vi "Viewer.vi"(4 "Col Array Refnum":refnum<vi>, 5 "RepoPath Refnum":refnum<vi>, 6 "SetList Layout Ref":refnum<vi>, 7 "GitCmd Refnum":refnum<vi>, 8 "SetList Dev queue":refnum<queue>, 9 "SetList VariableManager ref":refnum<vi>, 10 "SetList Clipboard ref":refnum<vi>) -> ()   [LabVIEW 2013]
doc: "View read-only procedure (table, variables, functions, device setup). Copy values from viewer into SetList via input references."
uses:
  DeviceVIs/Device/Device.lvclass
  ColumnVIs/Column/Column.lvclass
  VariableManagerCodes/VariableManager/VariableManager.lvclass
  <vilib>/Utility/miscctls.llb/LVRowAndColumnTypeDef.ctl
  VariableManagerCodes/API/VariableManagerAPI.lvlib
panel:
  in  "LoadFromRepo":bool
  out "SetList Procedure Description":string
  out "SetList Hash":string
  out "Invalid ref Warning":string="LOST LINK TO SetList:\nPlease close this window and relaunch from SetList."
  out "SetList Procedure Name":string
  out "SetList Version":string
  in  "Tab Control":T1(tab)
  in  "Layouts2SetList Button":bool
  in  "FitCol2Text Button":bool
  in  "View Devices Button":bool
  in  "Select Layout":i32(ring)=-1 items=["(On-the-fly)"=-2, "All"=-1]
  in  "Viewer Table":string[][](table)=[["", "", "Ramp", "1", "0.1", "0", "0", "0", "0", "0", "0", "0", "0", "0", "0", "0", "0", "0", "0", "0", "0", "0", "0", "0", "0", "0", "0", "0", "0", "0"]]
  out "Useful Functions":string="-- not functionality for strings (always treated as double)\nfunction bnot(a)\n   -- this \"(bool exp.) and b or c\" is equivalent to \"(bool exp.) ? b : c\" syntax.\n   -- caution: undefined variables evaluate to \"false\" so will NOT throw an error as argument\n   return a==0 and 1 or 0\nend"
  out "Viewer: User Functions":string
  out "RepoPath?":bool
  out "GitCmd?":bool
  out "SetList Col Array?":bool
  out "SetList Layout Ring?":bool
  out "SetList Dev queue?":bool
  out "SetList Variables?\n(on startup only)":bool
  out "SetList Clipboard?":bool
  in  "Viewer VariableManager.lvclass":refnum<class "VariableManager.lvclass">
  out "View Dev queue":refnum<queue>
  out "View Col array":refnum<class "Column.lvclass">[](array[class])
  in  "Devices":refnum<class "Device.lvclass">[](array[class])
  out "Mouse Down on header":bool
  # "SetList Viewer (Read-only)"
  # "In the context of ramps several variables are passed or specified that may be used here:\n\n   - f the fractional position of a point in a ramp\n   - t the current time in a ramp\n   - dt the current timestep size.\n   - tMax the total duration of the ramp"
  # "Invalid reference?"
  # "SetList references"
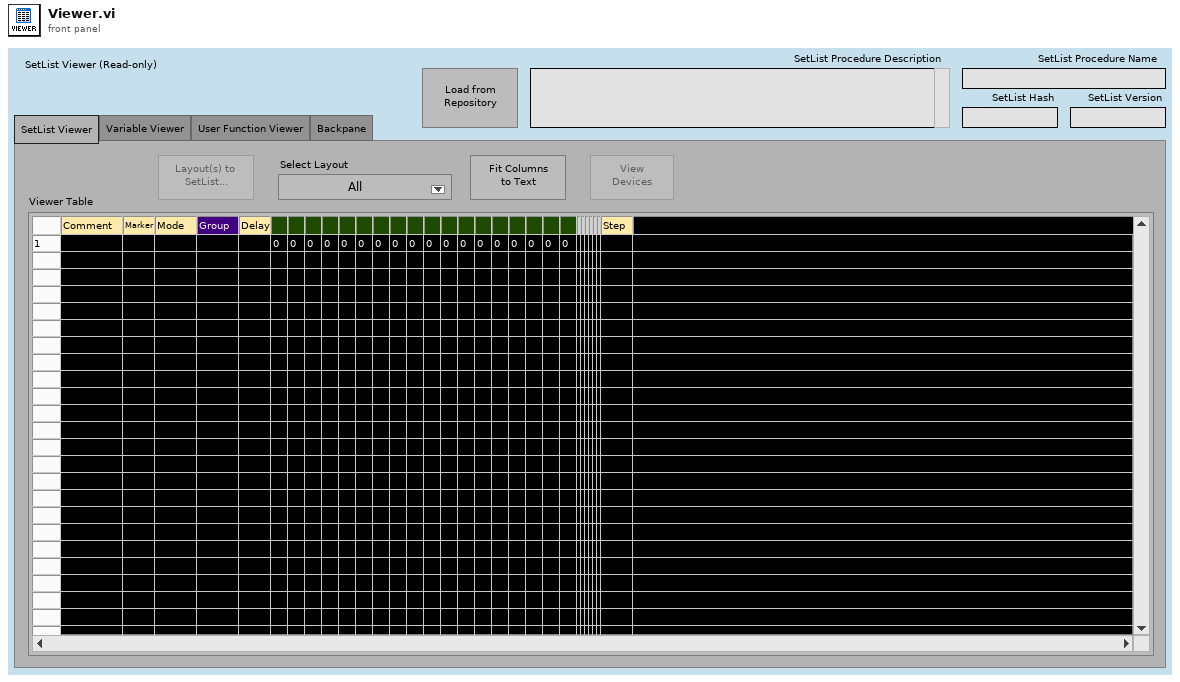
[diagram p1: front panel]
types:
  T1 = enum32{"SetList Viewer", "Variable Viewer", "User Function Viewer", "Backpane"}
  T2 = typedef "LVRowAndColumnTypeDef.ctl" = cluster{"Row":i32, "Column":i32}
  T3 = enum8{"Enabled", "Disabled", "Disabled and Grayed Out"}
  T4 = typedef "SaveCluster.ctl" = cluster{"Version":string, "Devices":refnum<class "Device.lvclass">[], "Select Layout":i32, "Layout:Strings And Values []":T5, "User defined functions":string, "VariableManager":refnum<class "VariableManager.lvclass">}
  T5 = typedef "LVStringsAndValuesArrayTypeDef_I32.ctl" = cluster{"String":string, "Value":i32}[]
  T6 = typedef "CommitCluster.ctl" = cluster{"Hash":string, "Date":string, "Name":string}
  T7 = typedef "LVPoint32TypeDef.ctl" = cluster{"Horizontal":i32, "Vertical":i32}
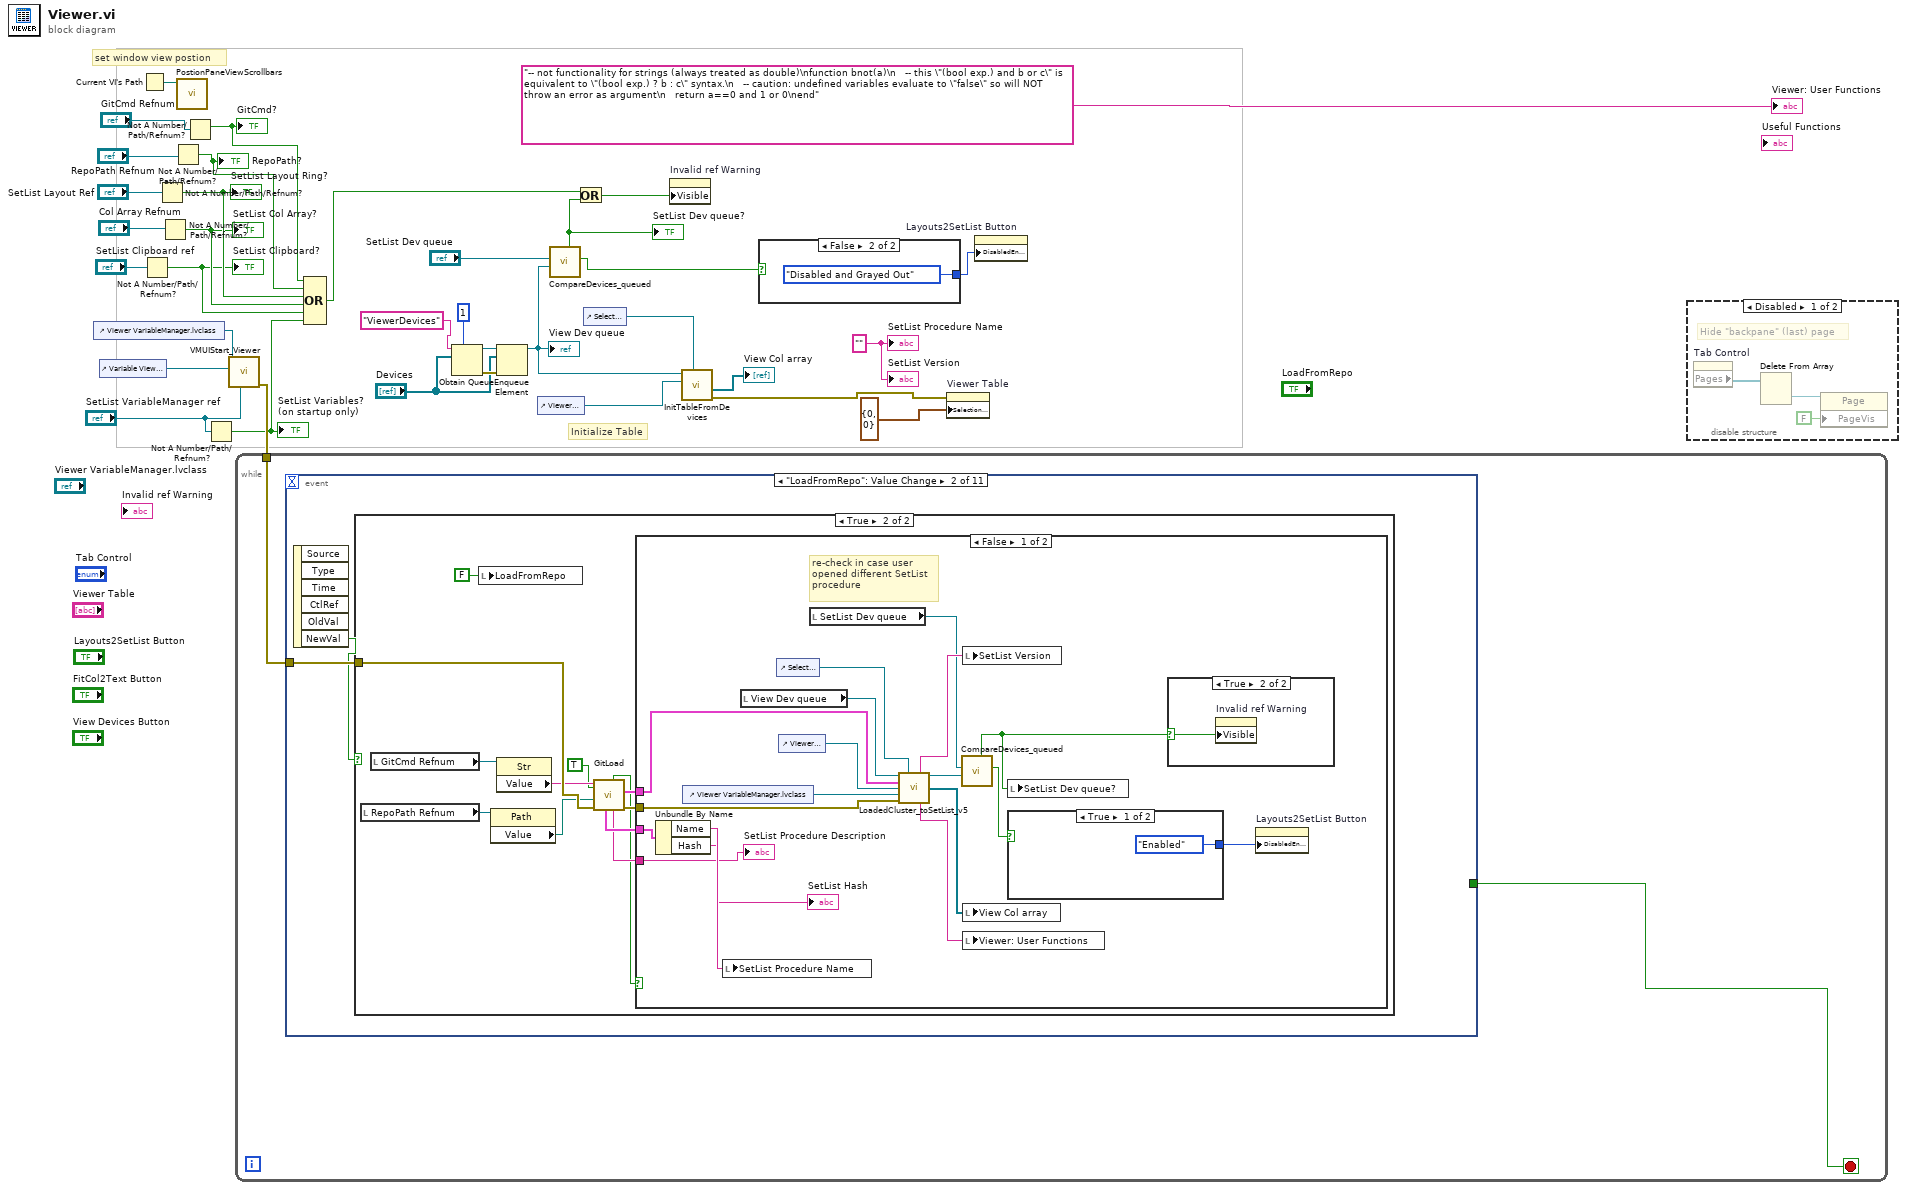
[diagram p0: block diagram]
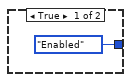
[diagram p2: hidden frame]
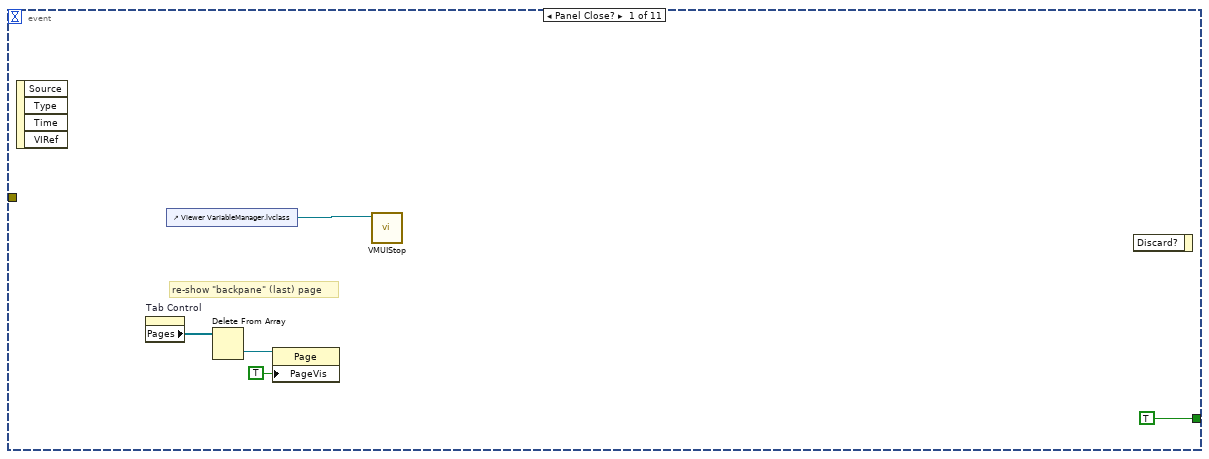
[diagram p4: hidden frame]
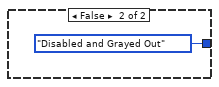
[diagram p7: hidden frame]
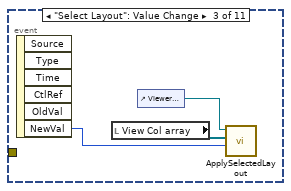
[diagram p9: hidden frame]
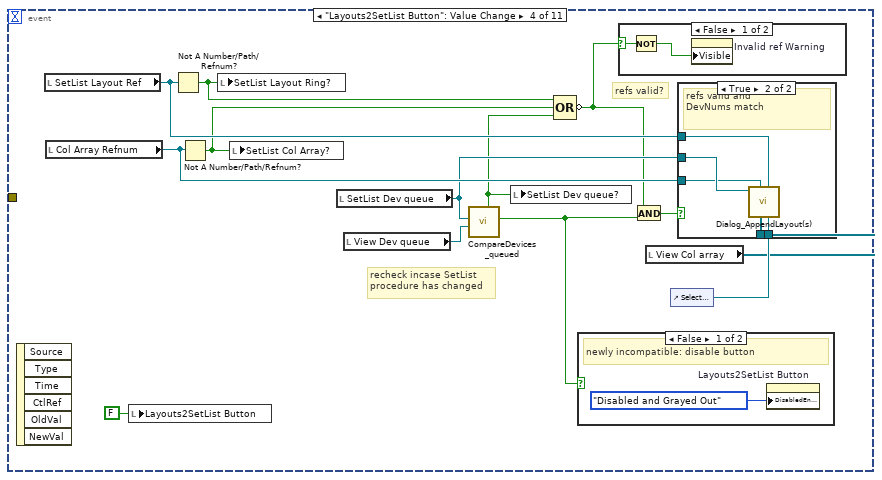
[diagram p10: hidden frame]
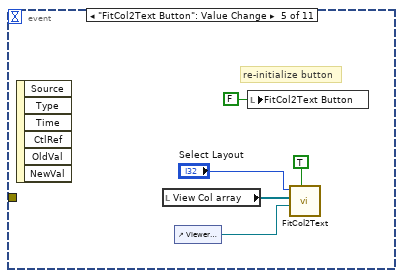
[diagram p14: hidden frame]
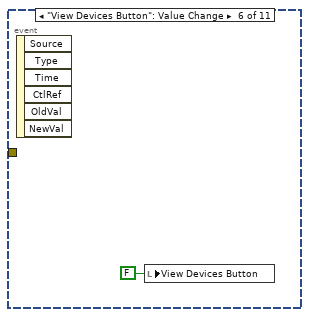
[diagram p15: hidden frame]
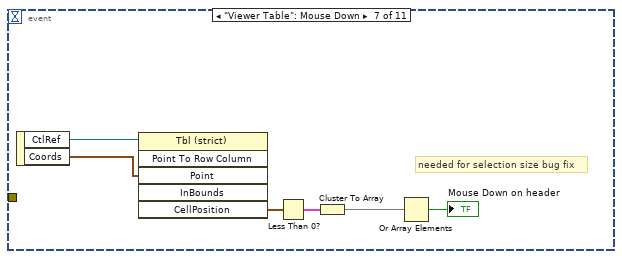
[diagram p16: hidden frame]
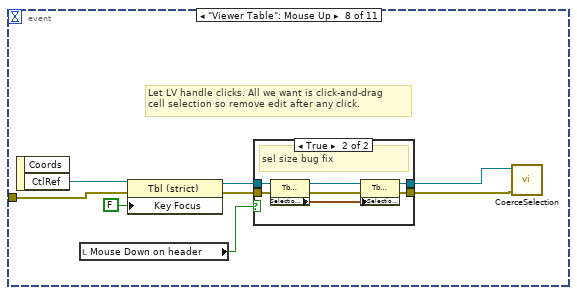
[diagram p17: hidden frame]
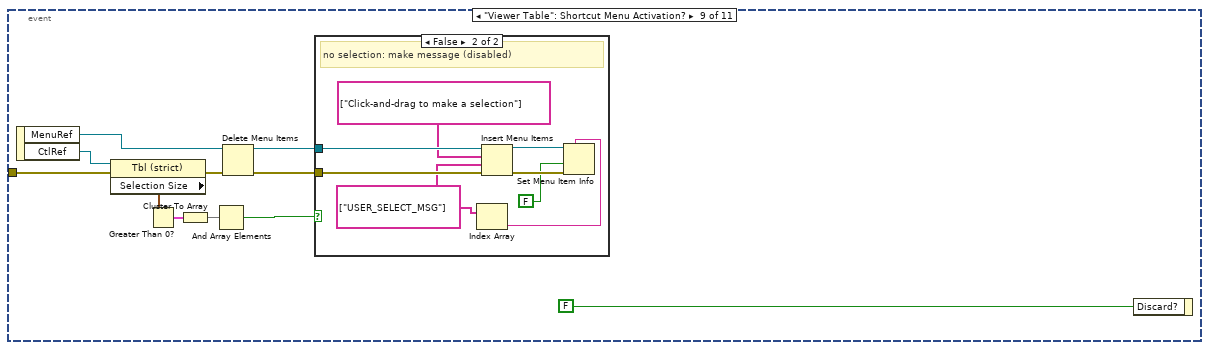
[diagram p19: hidden frame]
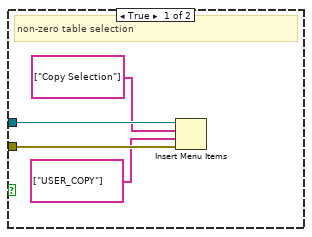
[diagram p20: hidden frame]
diagram:
  w27 = "" ("SetList Procedure Name")
  # "set window view postion"
  # "Initialize Table"
  n1 = control-ref of="Viewer VariableManager.lvclass"() -> (w24:refnum<vi>)
  n2 = control-ref of="Variable View Pane"() -> (w25:refnum<vi>)
  n3 = Current VI's Path() -> (path=w18:path)
  n4 = Not A Number/Path/Refnum?(number/path/refnum="SetList Clipboard ref") -> (NaN/Path/Refnum?=w13:bool)
  "SetList Clipboard?" <- w13
  n5 = Not A Number/Path/Refnum?(number/path/refnum="SetList Layout Ref") -> (NaN/Path/Refnum?=w15:bool)
  "SetList Layout Ring?" <- w15
  n6 = Not A Number/Path/Refnum?(number/path/refnum="Col Array Refnum") -> (NaN/Path/Refnum?=w14:bool)
  "SetList Col Array?" <- w14
  n7 = Not A Number/Path/Refnum?(number/path/refnum="RepoPath Refnum") -> (NaN/Path/Refnum?=w1:bool)
  "RepoPath?" <- w1
  n8 = call "PostionPaneViewScrollbars.vi"("vi path"=w18) -> ()  [unwired: 10 in, 1 out]
  n9 = Not A Number/Path/Refnum?(number/path/refnum="GitCmd Refnum") -> (NaN/Path/Refnum?=w2:bool)
  "GitCmd?" <- w2
  n10 = Not A Number/Path/Refnum?(number/path/refnum="SetList VariableManager ref") -> (NaN/Path/Refnum?=w12:bool)
  "SetList Variables?\n(on startup only)" <- w12
  n11 = call "VMUIStart_Viewer.vi"("SetList VariableManager Ref in"="SetList VariableManager ref", "SubPanelRef"=w25, "Viewer VariableManager Ref in"=w24) -> ("error out"=w23:errorcluster)  [unwired: 7 in, 1 out]
  n12 = while {
    tunnel: w23 -> [w36]
    stop <- w37 stop-if-true
    n13 = event shown="[1] \"LoadFromRepo\": Value Change" {
      selector: _ -> [_ _ _ _ _ _ _ _ _ _ _]
      dyn-events: _ -> [_ _ _ _ _ _ _ _ _ _ _]
      timeout: _ -> [_ _ _ _ _ _ _ _ _ _ _]
      tunnel: [TRUE ("true") _ _ _ _ _ _ _ _ _ _] -> w37
      tunnel: w36 -> [_ w44 _ _ _ _ _ w120 w141 w155 _]
      event Panel Close? {
        # "re-show \"backpane\" (last) page"
        n14 = event-data() -> ()  [unwired: 1 in, 4 out]
        n15 = property on="Tab Control" class="TabCtl (strict)"() -> ("Pages"=w40:refnum<vi>[])  [unwired: 2 in, 2 out]
        n16 = control-ref of="Viewer VariableManager.lvclass"() -> (w41:refnum<vi>)
        n17 = Delete From Array(array=w40) -> (deleted portion=w39:refnum<vi>)  [unwired: 2 in, 1 out]
        n18 = property class="Page"(reference=w39, "PageVis"=TRUE ("Page Visible")) -> ()  [unwired: 1 in, 2 out]
        n19 = call "VMUIStop.vi"("VariableManagerRef in"=w41) -> ()  [unwired: 9 in, 2 out]
        n20 = event-data() -> ()  [unwired: 2 in, 1 out]
      }
      event "LoadFromRepo": Value Change {
        n21 = event-data() -> ("NewVal"=w43:bool)  [unwired: 1 in, 5 out]
        n22 = case shown="True" w43 {
          tunnel: w44 -> [_ w54]
          frame False {
          }
          frame True {
            n23 = local read "RepoPath Refnum"() -> (w50:refnum<vi>)
            n24 = local read "GitCmd Refnum"() -> (w52:refnum<vi>)
            n25 = local write "LoadFromRepo"(FALSE ("LoadFromRepo")) -> ()
            n26 = property class="Path"(reference=w50) -> ("Value"=w49:path)  [unwired: 1 in, 2 out]
            n27 = property class="Str"(reference=w52) -> ("Value"=w51:string)  [unwired: 1 in, 2 out]
            n28 = call "GitLoad.vi"("Viewer?"=TRUE, "error in (no error)"=w54, "Directory"=w49, "Git exec"=w51) -> ("error out"=w55:errorcluster, "Save Cluster"=w56:T4, "Loaded Description"=w47:string, "User Cancelled"=w45:bool, "Loaded Commit Info"=w53:T6)  [unwired: 1 in, 2 out]
            n29 = case shown="False" w45 {
              tunnel: w56 -> [w62 _]
              tunnel: w55 -> [w61 _]
              tunnel: w53 -> [w60 _]
              tunnel: w47 -> [w58 _]
              frame False {
                # "re-check in case user\nopened different SetList\nprocedure"
                n30 = Unbundle By Name(w60) -> ("Name"=w59:string, "Hash"=→"SetList Hash":string)
                n31 = control-ref of="Viewer VariableManager.lvclass"() -> (w69:refnum<vi>)
                n32 = local write "SetList Procedure Name"(w59) -> ()
                n33 = local read "View Dev queue"() -> (w65:refnum<queue>)
                n34 = control-ref of="Select Layout"() -> (w74:refnum<vi>)
                n35 = control-ref of="Viewer Table"() -> (w73:refnum<vi>)
                n36 = local read "SetList Dev queue"() -> (w67:refnum<queue>)
                n37 = call "LoadedCluster_toSetList_v5.vi"("Devices queue"=w65, "Layout Ref"=w74, "Save Cluster"=w62, "Table Ref in"=w73, "VariableManagerRef"=w69, "error in (no error)"=w61) -> ("Loaded Version"=w72:string, "Devices queue out"=w63:refnum<queue>, "Col array"=w71:refnum<class "Column.lvclass">[], "User defined functions"=w70:string)  [unwired: 4 in, 2 out]
                n38 = call "CompareDevices_queued.vi"("New Dev queue"=w63, "Old Dev queue"=w67) -> ("compatible?"=w66:bool, "Old Dev queue invalid?"=w64:bool)  [unwired: 7 in, 1 out]
                n39 = local write "SetList Version"(w72) -> ()
                n40 = local write "View Col array"(w71) -> ()
                n41 = local write "Viewer: User Functions"(w70) -> ()
                n42 = local write "SetList Dev queue?"(w64) -> ()
                n43 = case shown="True" w66 {
                  tunnel: [T3."Enabled" ("Disabled") T3."Disabled and Grayed Out" ("Disabled")] -> w68
                  frame True {
                  }
                  frame False {
                  }
                }
                n44 = case shown="True" w64 {
                  selector: w64 -> [_ w75]
                  frame False {
                  }
                  frame True {
                    n45 = property on="Invalid ref Warning" class="Str"("Visible"=w75) -> ()  [unwired: 2 in, 2 out]
                  }
                }
                n46 = property on="Layouts2SetList Button" class="Bool (strict)"("DisabledEnum"=w68) -> ()  [unwired: 2 in, 2 out]
                "SetList Procedure Description" <- w58
              }
              frame True {
              }
            }
          }
        }
      }
      event "Select Layout": Value Change {
        n47 = event-data() -> ("NewVal"=w80:i32)  [unwired: 1 in, 5 out]
        n48 = local read "View Col array"() -> (w79:refnum<class "Column.lvclass">[])
        n49 = control-ref of="Viewer Table"() -> (w78:refnum<vi>)
        n50 = call "ApplySelectedLayout.vi"("Layout index"=w80, "Col array"=w79, "Tbl Refnum"=w78) -> ()  [unwired: 8 in, 1 out]
      }
      event "Layouts2SetList Button": Value Change {
        # "recheck incase SetList\nprocedure has changed"
        # "refs valid?"
        n51 = event-data() -> ()  [unwired: 1 in, 6 out]
        n52 = local read "SetList Layout Ref"() -> (w91:refnum<vi>)
        n53 = local read "Col Array Refnum"() -> (w86:refnum<vi>)
        n54 = local write "Layouts2SetList Button"(FALSE ("Layouts2SetList Button")) -> ()
        n55 = Not A Number/Path/Refnum?(number/path/refnum=w91) -> (NaN/Path/Refnum?=w90:bool)
        n56 = Not A Number/Path/Refnum?(number/path/refnum=w86) -> (NaN/Path/Refnum?=w87:bool)
        n57 = local write "SetList Layout Ring?"(w90) -> ()
        n58 = local write "SetList Col Array?"(w87) -> ()
        n59 = local read "SetList Dev queue"() -> (w84:refnum<queue>)
        n60 = local read "View Dev queue"() -> (w85:refnum<queue>)
        n61 = call "CompareDevices_queued.vi"("New Dev queue"=w85, "Old Dev queue"=w84) -> ("compatible?"=w82:bool, "Old Dev queue invalid?"=w83:bool)  [unwired: 7 in, 1 out]
        n62 = local write "SetList Dev queue?"(w83) -> ()
        n63 = Compound Arithmetic op=OR(w90, w87, w83) -> (invert w81:bool)
        n64 = case shown="False" w82 {
          frame False {
            # "newly incompatible: disable button"
            n65 = property on="Layouts2SetList Button" class="Bool (strict)"("DisabledEnum"=T3."Disabled and Grayed Out" ("Disabled")) -> ()  [unwired: 2 in, 2 out]
          }
          frame True {
          }
        }
        n66 = case shown="False" w81 {
          selector: w81 -> [w95 _]
          frame False {
            n67 = Not(x=w95) -> (.not. x?=w94:bool)
            n68 = property on="Invalid ref Warning" class="Str"("Visible"=w94) -> ()  [unwired: 2 in, 2 out]
          }
          frame True {
          }
        }
        n69 = And(x=w81, y=w82) -> (x .and. y?=w92:bool)
        n70 = local read "View Col array"() -> (w88:refnum<class "Column.lvclass">[])
        n71 = control-ref of="Select Layout"() -> (w89:refnum<vi>)
        n72 = case shown="True" w92 {
          tunnel: w91 -> [_ w101]
          tunnel: w84 -> [_ w98]
          tunnel: w89 -> [_ w100]
          tunnel: w88 -> [_ w99]
          tunnel: w86 -> [_ w97]
          frame False {
            # "refs inalid or\nDevNum mis-match"
          }
          frame True {
            # "refs valid and \nDevNums match"
            n73 = call "Dialog_AppendLayout(s).vi"("Viewer Layout Ref"=w100, "SetList Layout Ref"=w101, "View Col array"=w99, "Col Array Refnum"=w97, "SetList Dev queue"=w98) -> ()  [unwired: 7 in]
          }
        }
      }
      event "FitCol2Text Button": Value Change {
        # "re-initialize button"
        n74 = event-data() -> ()  [unwired: 1 in, 6 out]
        n75 = local read "View Col array"() -> (w106:refnum<class "Column.lvclass">[])
        n76 = control-ref of="Viewer Table"() -> (w103:refnum<vi>)
        n77 = local write "FitCol2Text Button"(FALSE ("FitCol2Text Button")) -> ()
        n78 = call "FitCol2Text.vi"("Defer Updates?"=TRUE, "SetList Table ref"=w103, "Col array"=w106, "Select Layout"="Select Layout") -> ()  [unwired: 7 in, 1 out]
      }
      event "View Devices Button": Value Change {
        n79 = event-data() -> ()  [unwired: 1 in, 6 out]
        n80 = local write "View Devices Button"(FALSE ("View Devices Button")) -> ()
      }
      event "Viewer Table": Mouse Down {
        # "needed for selection size bug fix"
        n81 = event-data() -> ("CtlRef"=w113:refnum<vi>, "Coords"=w112:T7)  [unwired: 1 in]
        n82 = invoke on="Invoke Node" class="Tbl (strict)" method="Point To Row Column"(reference=w113, "Point"=w112) -> ("CellPosition"=w111:T2)  [unwired: 4 in, 5 out]
        n83 = Less Than 0?(x=w111) -> (x < 0?=w110:cluster{"Row":bool, "Column":bool})
        n84 = Cluster To Array(cluster=w110) -> (array=w109:bool[])
        n85 = Or Array Elements(Boolean array=w109) -> (logical OR=→"Mouse Down on header":bool)
      }
      event "Viewer Table": Mouse Up {
        # "Let LV handle clicks. All we want is click-and-drag\ncell selection so remove edit after any click."
        n86 = event-data() -> ("CtlRef"=w121:refnum<vi>)  [unwired: 1 in, 1 out]
        n87 = local read "Mouse Down on header"() -> (w114:bool)
        n88 = property class="Tbl (strict)"(reference=w121, error in=w120, "Key Focus"=FALSE) -> (reference out=w118:refnum<vi>, error out=w116:errorcluster)
        n89 = case shown="True" w114 {
          tunnel: w118 -> [w123 w127]
          tunnel: [w123 w126] -> w117
          tunnel: w116 -> [w122 w125]
          tunnel: [w122 w124] -> w115
          frame False {
          }
          frame True {
            # "sel size bug fix"
            n90 = property on="Property Node" class="Tbl (strict)"(reference=w127, error in=w125) -> (reference out=w128:refnum<vi>, error out=w130:errorcluster, "Selection Start"=w129:T2)
            n91 = property on="Property Node" class="Tbl (strict)"(reference=w128, error in=w130, "Selection Start"=w129) -> (reference out=w126:refnum<vi>, error out=w124:errorcluster)
          }
        }
        n92 = call "CoerceSelection.vi"("error in (no error)"=w115, "SetList Table ref"=w117) -> ()  [unwired: 9 in, 1 out]
      }
      event "Viewer Table": Shortcut Menu Activation? {
        n93 = event-data() -> ("MenuRef"=w134:refnum<k9>, "CtlRef"=w140:refnum<vi>)  [unwired: 1 in]
        n94 = property class="Tbl (strict)"(reference=w140, error in=w141) -> (error out=w136:errorcluster, "Selection Size"=w139:T2)  [unwired: 1 out]
        n95 = Greater Than 0?(x=w139) -> (x > 0?=w138:cluster{"Row":bool, "Column":bool})
        n96 = Cluster To Array(cluster=w138) -> (array=w137:bool[])
        n97 = And Array Elements(Boolean array=w137) -> (logical AND=w132:bool)
        n98 = Delete Menu Items(6:w136, 9:w134) -> (0:w135:errorcluster, 3:w133:refnum<k9>)  [unwired: 2 in]
        n99 = case shown="False" w132 {
          tunnel: w135 -> [w145 w153]
          tunnel: w133 -> [w144 w152]
          frame True {
            # "non-zero table selection"
            n100 = Insert Menu Items(6:w145, 7:string[] ["USER_COPY"] ("item names"), 8:string[] ["Copy Selection"] ("item names"), 9:w144) -> ()  [unwired: 2 in, 3 out]
          }
          frame False {
            w148 = string[] ["USER_SELECT_MSG"] ("item names")
            # "no selection: make message (disabled)"
            n101 = Index Array(array=w148) -> (element=w147:string)  [unwired: 1 in]
            n102 = Insert Menu Items(6:w153, 7:w148, 8:string[] ["Click-and-drag to make a selection"] ("item names"), 9:w152) -> (0:w151:errorcluster, 3:w146:refnum<k9>)  [unwired: 2 in, 1 out]
            n103 = Set Menu Item Info(7:w147, 8:w151, 9:FALSE ("enabled"), 11:w146) -> ()  [unwired: 3 in, 2 out]
          }
        }
        n104 = event-data("Discard?"=FALSE) -> ()  [unwired: 1 in, 1 out]
      }
      event "Viewer Table": Shortcut Menu Selection (User) {
        n105 = event-data() -> ("CtlRef"=w154:refnum<vi>, "ItemTag"=w156:string)  [unwired: 1 in]
        n106 = case shown="\"USER_COPY\"" w156 {
          tunnel: w155 -> [_ w160]
          tunnel: w154 -> [_ w159]
          frame Default {
          }
          frame "USER_COPY" {
            n107 = local read "SetList Clipboard ref"() -> (w157:refnum<vi>)
            n108 = Not A Number/Path/Refnum?(number/path/refnum=w157) -> (NaN/Path/Refnum?=w158:bool)
            n109 = case shown="True" w158 {
              selector: w158 -> [_ w164]
              tunnel: w160 -> [w163 _]
              tunnel: w159 -> [w162 _]
              tunnel: w157 -> [w161 _]
              frame False {
                # "valid refunm"
                n110 = call "CopySelectedCells.vi"("Clipboard"=w161, "error in (no error)"=w163, "Table CtlRef In"=w162) -> ()  [unwired: 7 in, 2 out]
              }
              frame True {
                # "invalid refnum"
                n111 = property on="Invalid ref Warning" class="Str"("Visible"=w164) -> ()  [unwired: 2 in, 2 out]
                n112 = property on="SetList Clipboard?" class="Bool (strict)"("Value"=w164) -> ()  [unwired: 2 in, 2 out]
              }
            }
          }
        }
      }
      event "Viewer Table": Value Change {
        # "no editing!\n(fixes type while holding mouse down bug)"
        n113 = event-data() -> ("OldVal"=w165:string[][])  [unwired: 1 in, 5 out]
        n114 = local write "Viewer Table"(w165) -> ()
      }
    }
  }
  n115 = Compound Arithmetic op=OR(w2, w1, w15, w14, w13, w12) -> (w8:bool)
  n116 = Obtain Queue(max queue size (-1, unlimited)=1, name (unnamed)="ViewerDevices", element data type="Devices") -> (queue out=w33:refnum<queue>, error out=w32:errorcluster)  [unwired: 2 in, 1 out]
  n117 = Enqueue Element(queue=w33, element="Devices", error in (no error)=w32) -> (queue out=w10:refnum<queue>)  [unwired: 1 in, 2 out]
  "View Dev queue" <- w10
  n118 = control-ref of="Viewer Table"() -> (w28:refnum<vi>)
  n119 = call "CompareDevices_queued.vi"("New Dev queue"=w10, "Old Dev queue"="SetList Dev queue") -> ("compatible?"=w6:bool, "Old Dev queue invalid?"=w9:bool)  [unwired: 7 in, 1 out]
  "SetList Dev queue?" <- w9
  n120 = Or(x=w8, y=w9) -> (x .or. y?=w5:bool)
  n121 = control-ref of="Select Layout"() -> (w29:refnum<vi>)
  n122 = property on="Invalid ref Warning" class="Str"("Visible"=w5) -> ()  [unwired: 2 in, 2 out]
  n123 = call "InitTableFromDevices.vi"("Layout Ref"=w29, "Table Ref in"=w28, "Devices queue"=w10) -> ("error out"=w21:errorcluster, "Col array"=→"View Col array":refnum<class "Column.lvclass">[])  [unwired: 5 in, 2 out]
  n124 = case shown="False" w6 {
    tunnel: [T3."Enabled" ("Disabled") T3."Disabled and Grayed Out" ("Disabled")] -> w7
    frame True {
    }
    frame False {
    }
  }
  n125 = property on="Viewer Table" class="Tbl (strict)"(error in=w21, "Selection Size"=T2 {"Row"=0, "Column"=0}) -> ()  [unwired: 1 in, 2 out]
  n126 = property on="Layouts2SetList Button" class="Bool (strict)"("DisabledEnum"=w7) -> ()  [unwired: 2 in, 2 out]
  n127 = disable-structure shown="Disabled" {
    frame Disabled {
      # "Hide \"backpane\" (last) page"
      n128 = property on="Tab Control" class="TabCtl (strict)"() -> ("Pages"=w168:refnum<vi>[])  [unwired: 2 in, 2 out]
      n129 = Delete From Array(array=w168) -> (deleted portion=w169:refnum<vi>)  [unwired: 2 in, 1 out]
      n130 = property class="Page"(reference=w169, "PageVis"=FALSE ("Page Visible")) -> ()  [unwired: 1 in, 2 out]
    }
    frame Enabled {
    }
  }
  "SetList Procedure Name" <- w27
  "SetList Version" <- w27
  "Viewer: User Functions" <- "-- not functionality for strings (always treated as double)\nfunction bnot(a)\n   -- this \"(bool exp.) and b or c\" is equivalent to \"(bool exp.) ? b : c\" syntax.\n   -- caution: undefined variables evaluate to \"false\" so will NOT throw an error as argument\n   return a==0 and 1 or 0\nend" ("Viewer: User Functions")
